vi "make_alarm_LCW.vi"(3 "enabled":bool=TRUE, 4 "WFS1_lolo":dbl=1.3, 5 "M123_lolo":dbl=0.3, 6 "WFS1_lo":dbl=1.6, 7 "M123_lo":dbl=0.6, 8 "time_last_alarm_in":timestamp, 11 "value_array":dbl[](array[numeric])) -> (0 "time_last_alarm_out":timestamp, 2 "alarm_status":u32(colorbox))   [LabVIEW 2019]
panel:
  out "message":string
  in  "interval":dbl=600.0
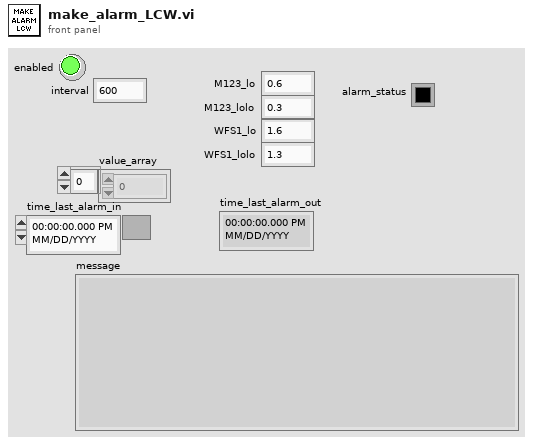
[diagram p1: front panel]
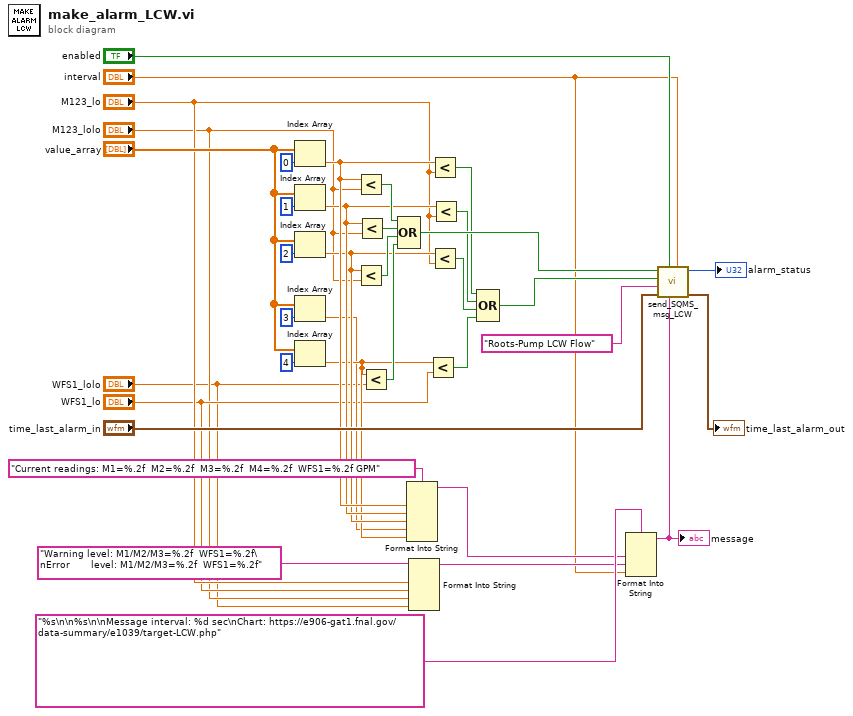
[diagram p0: block diagram]
diagram:
  n1 = Index Array(array="value_array", index=0) -> (element=w16:dbl)
  n2 = Index Array(array="value_array", index=1) -> (element=w15:dbl)
  n3 = Index Array(array="value_array", index=2) -> (element=w14:dbl)
  n4 = Index Array(array="value_array", index=3) -> (element=w12:dbl)
  n5 = Index Array(array="value_array", index=4) -> (element=w13:dbl)
  n6 = Less?(x=w16, y="M123_lolo") -> (x < y?=w33:bool)
  n7 = Less?(x=w14, y="M123_lolo") -> (x < y?=w31:bool)
  n8 = Less?(x=w15, y="M123_lolo") -> (x < y?=w32:bool)
  n9 = Less?(x=w13, y="WFS1_lolo") -> (x < y?=w30:bool)
  n10 = Compound Arithmetic op=OR(w33, w32, w31, w30) -> (w28:bool)
  n11 = Format Into String(format string="Current readings: M1=%.2f  M2=%.2f  M3=%.2f  M4=%.2f  WFS1=%.2f GPM" ("msg"), w16, w15, w14, w12, w13) -> (resulting string=w5:string)  [unwired: 2 in, 1 out]
  n12 = Format Into String(format string="Warning level: M1/M2/M3=%.2f  WFS1=%.2f\nError       level: M1/M2/M3=%.2f  WFS1=%.2f" ("msg"), "M123_lo", "WFS1_lo", "M123_lolo", "WFS1_lolo") -> (resulting string=w4:string)  [unwired: 2 in, 1 out]
  n13 = Less?(x=w13, y="WFS1_lo") -> (x < y?=w24:bool)
  n14 = Less?(x=w16, y="M123_lo") -> (x < y?=w27:bool)
  n15 = Less?(x=w14, y="M123_lo") -> (x < y?=w25:bool)
  n16 = Less?(x=w15, y="M123_lo") -> (x < y?=w26:bool)
  n17 = Compound Arithmetic op=OR(w27, w26, w25, w24) -> (w23:bool)
  n18 = Format Into String(format string="%s\n\n%s\n\nMessage interval: %d sec\nChart: https://e906-gat1.fnal.gov/data-summary/e1039/target-LCW.php" ("msg"), w5, w4, "interval") -> (resulting string=w2:string)  [unwired: 2 in, 1 out]
  "message" <- w2
  n19 = call "send_SQMS_msg_LCW.vi"("alarm_interval"="interval", "msg"=w2, "enabled"="enabled", "time_last_alarm_in"="time_last_alarm_in", "title"="Roots-Pump LCW Flow", "warning"=w23, "error"=w28) -> ("time_last_alarm_out"=→"time_last_alarm_out":timestamp, "alarm_status"=→"alarm_status":u32)  [unwired: 2 in, 1 out]
